vi "HOLD.vi"() -> ()   [LabVIEW 2015]
uses:
  Global.vi
panel:
  out "Options":string
  in  "Hold":bool
  in  "stop":bool
  out "VAR index":i32
  out "Val":string
  out "Old_Val":string
  out "Set":bool
  out "Recieved":bool
  in  "Var":string="HOLD"
  # "Wait for user input.\n\nValue Type: STR\nOptions: None"
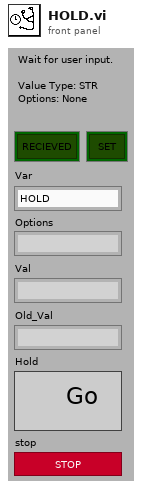
[diagram p1: front panel]
types:
  T1 = typedef "Semaphore RefNum" = refnum<k1>
  T2 = cluster{"VAR":string, "Options":string, "Val":string, "Recieved":bool, "Set":bool}[]
  T3 = cluster{"VAR":string, "Options":string, "Val":string, "Recieved":bool, "Set":bool}
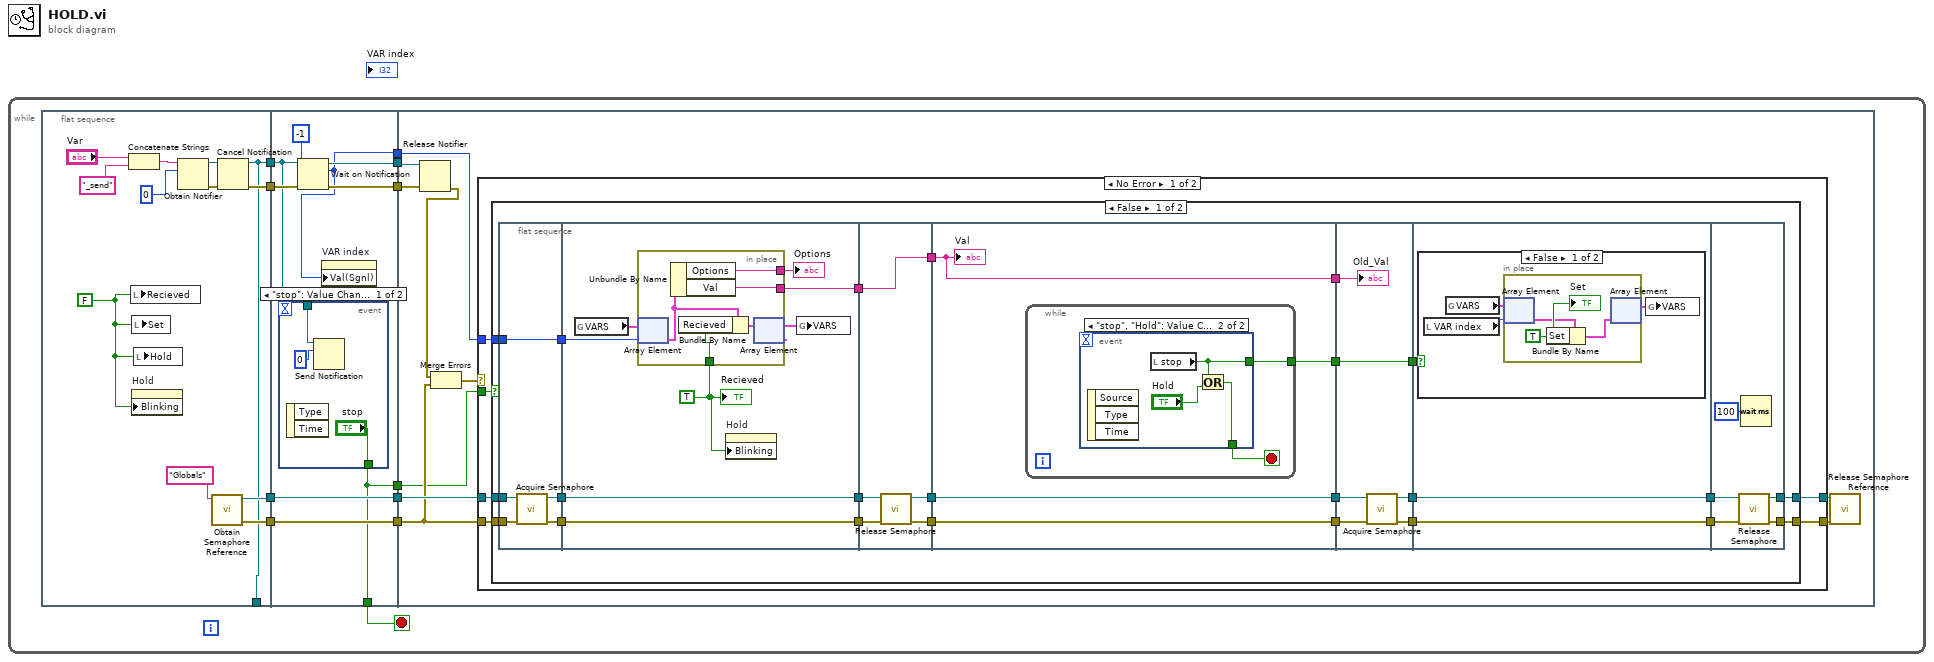
[diagram p0: block diagram]
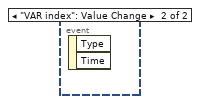
[diagram p2: hidden frame]
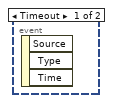
[diagram p3: hidden frame]
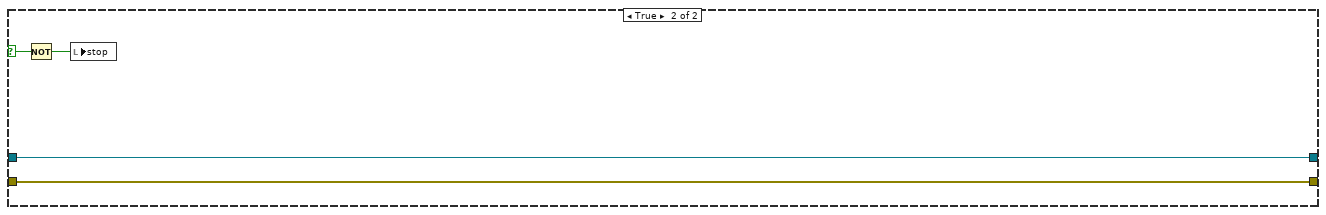
[diagram p5: hidden frame]
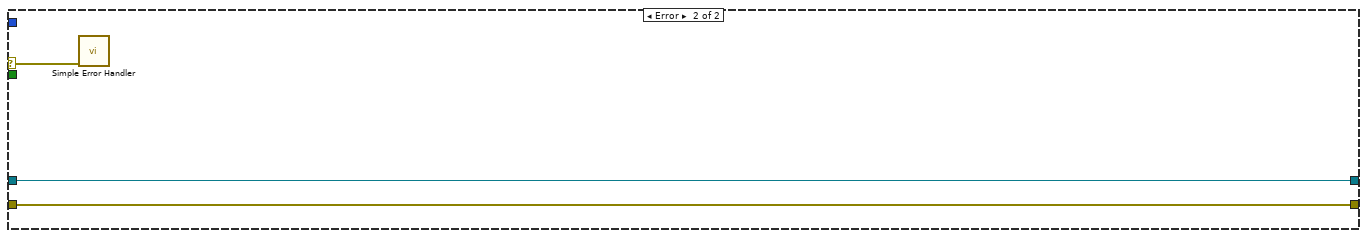
[diagram p6: hidden frame]
diagram:
  n1 = while {
    stop <- w2 stop-if-true
    n2 = flat-sequence {
      tunnel: [w14] -> w11
      tunnel: [w13] -> w10
      tunnel: [w22] -> w6
      tunnel: [w21] -> w4
      tunnel: [w13] -> _
      tunnel: w11 -> [w31]
      tunnel: w10 -> [w25]
      tunnel: [w30] -> w9
      tunnel: [w27] -> w8
      tunnel: [w26] -> w7
      tunnel: w6 -> [w29]
      tunnel: [w29] -> w5
      tunnel: w4 -> [w28]
      tunnel: [w28] -> w3
      tunnel: [w24] -> w2
      tunnel: [w24] -> w1
      tunnel: w9 -> [w38]
      tunnel: w8 -> [w39]
      tunnel: w7 -> [w45]
      tunnel: w5 -> [w44]
      tunnel: w3 -> [w41]
      tunnel: w1 -> [w36]
      frame #0 {
        w16 = FALSE ("notification")
        n3 = Concatenate Strings("Var", "_send") -> (w19:string)
        n4 = local write "Recieved"(w16) -> ()
        n5 = local write "Set"(w16) -> ()
        n6 = property on="Hold" class="Bool (strict)"("Blinking"=w16) -> ()  [unwired: 2 in, 2 out]
        n7 = local write "Hold"(w16) -> ()
        n8 = Obtain Notifier(name (unnamed)=w19, notification data type=0) -> (notifier out=w12:refnum<notifier>, error out=w15:errorcluster)  [unwired: 2 in, 1 out]
        n9 = call <vilib>:"Obtain Semaphore Reference.vi"("name (unnamed)"="Globals") -> ("error out"=w21:errorcluster, "semaphore"=w22:T1)  [unwired: 4 in, 1 out]
        n10 = Cancel Notification(0:w12, 3:w15) -> (8:w13:refnum<notifier>, 11:w14:errorcluster)  [unwired: 1 out]
      }
      frame #1 {
        n11 = event shown="[0] \"stop\": Value Change" {
          selector: _ -> [_ _]
          dyn-events: _ -> [_ _]
          timeout: _ -> [_ _]
          tunnel: ["stop" _] -> w24
          tunnel: w25 -> [w34 _]
          event "stop": Value Change {
            n12 = event-data() -> ()  [unwired: 1 in, 2 out]
            n13 = Send Notification(notification=0, notifier=w34) -> ()  [unwired: 1 in, 2 out]
          }
          event "VAR index": Value Change {
            n14 = event-data() -> ()  [unwired: 1 in, 2 out]
          }
        }
        n15 = Wait on Notification(notifier=w25, timeout in ms (-1)=-1, error in (no error)=w31) -> (notifier out=w30:refnum<notifier>, notification=w26:i32, error out=w27:errorcluster)  [unwired: 1 in, 1 out]
        n16 = property on="VAR index" class="DigNum (strict)"("Val(Sgnl)"=w26) -> ()  [unwired: 2 in, 2 out]
      }
      frame #2 {
        n17 = Release Notifier(notifier=w38, error in (no error)=w39) -> (error out=w37:errorcluster)  [unwired: 1 in, 2 out]
        n18 = Merge Errors(w37, w41) -> (w40:errorcluster)
        n19 = case shown="No Error" w40 {
          selector: w40 -> [_ w131]
          tunnel: w45 -> [w51 _]
          tunnel: w44 -> [w50 w133]
          tunnel: w41 -> [w49 w132]
          tunnel: [w48 w132] -> w43
          tunnel: [w47 w133] -> w42
          tunnel: w36 -> [w46 _]
          frame No Error {
            n20 = case shown="False" w46 {
              selector: w46 -> [_ w128]
              tunnel: w51 -> [w59 _]
              tunnel: w50 -> [w58 w130]
              tunnel: w49 -> [w57 w129]
              tunnel: [w56 w129] -> w48
              tunnel: [w55 w130] -> w47
              frame False {
                n21 = flat-sequence {
                  tunnel: w57 -> [w77]
                  tunnel: w58 -> [w78]
                  tunnel: w59 -> [w79]
                  tunnel: [w79] -> w74
                  tunnel: [w76] -> w73
                  tunnel: [w75] -> w72
                  tunnel: w74 -> [w83]
                  tunnel: w73 -> [w86]
                  tunnel: w72 -> [w87]
                  tunnel: [w87] -> w71
                  tunnel: [w86] -> w70
                  tunnel: [w82] -> w69
                  tunnel: w71 -> [w96]
                  tunnel: w70 -> [w97]
                  tunnel: [w95] -> w68
                  tunnel: [w94] -> w67
                  tunnel: [w93] -> w66
                  tunnel: w69 -> [w93]
                  tunnel: w68 -> [w101]
                  tunnel: w67 -> [w100]
                  tunnel: [w101] -> w65
                  tunnel: [w100] -> w64
                  tunnel: w66 -> [w98]
                  tunnel: [w99] -> w53
                  tunnel: [w98] -> w52
                  tunnel: w65 -> [w112]
                  tunnel: w64 -> [w109]
                  tunnel: [w111] -> w63
                  tunnel: [w110] -> w62
                  tunnel: [w108] -> w54
                  tunnel: w53 -> [w108]
                  tunnel: w52 -> [w107]
                  tunnel: [w115] -> w61
                  tunnel: w63 -> [w115]
                  tunnel: [w114] -> w60
                  tunnel: w62 -> [w114]
                  tunnel: w54 -> [w113]
                  tunnel: w61 -> [w126]
                  tunnel: w60 -> [w125]
                  tunnel: [w124] -> w56
                  tunnel: [w123] -> w55
                  frame #0 {
                    n22 = call <vilib>:"Acquire Semaphore.vi"("error in (no error)"=w77, "semaphore"=w78) -> ("error out"=w76:errorcluster, "semaphore out"=w75:T1)  [unwired: 3 in, 1 out]
                  }
                  frame #1 {
                    w81 = TRUE ("Found")
                    n23 = global read "Global.vi" "VARS"() -> (w84:T2)
                    n24 = in-place {
                      in-place-border: [w90] -> w82
                      in-place-border: w81 -> [w89]
                      in-place-border: [w88] -> w80
                      n25 = in-place-array #1(w84, w83) -> (w92:T3)
                      n26 = Unbundle By Name(w92) -> ("Options"=w88:string, "Val"=w90:string)
                      n27 = Bundle By Name(cluster=w92, "Recieved"=w89) -> (w91:T3)
                      n28 = in-place-array #1(w91) -> (w85:T2)  [unwired: 1 out]
                    }
                    "Options" <- w80
                    n29 = property on="Hold" class="Bool (strict)"("Blinking"=w81) -> ()  [unwired: 2 in, 2 out]
                    n30 = global write "Global.vi" "VARS"(w85) -> ()
                    "Recieved" <- w81
                  }
                  frame #2 {
                    n31 = call <vilib>:"Release Semaphore.vi"("error in (no error)"=w97, "semaphore"=w96) -> ("error out"=w94:errorcluster, "semaphore out"=w95:T1)  [unwired: 4 in]
                  }
                  frame #3 {
                    n32 = while {
                      tunnel: [w102] -> w99
                      stop <- w103 stop-if-true
                      n33 = event shown="[1] \"stop\", \"Hold\": Value Change" {
                        selector: _ -> [_ _]
                        dyn-events: _ -> [_ _]
                        timeout: _ -> [_ _]
                        tunnel: [_ w105] -> w103
                        tunnel: [_ w104] -> w102
                        event Timeout {
                          n34 = event-data() -> ()  [unwired: 1 in, 3 out]
                        }
                        event "stop", "Hold": Value Change {
                          n35 = event-data() -> ()  [unwired: 1 in, 3 out]
                          n36 = local read "stop"() -> (w104:bool)
                          n37 = Or(x=w104, y="Hold") -> (x .or. y?=w105:bool)
                        }
                      }
                    }
                    "Val" <- w98
                  }
                  frame #4 {
                    n38 = call <vilib>:"Acquire Semaphore.vi"("error in (no error)"=w109, "semaphore"=w112) -> ("error out"=w110:errorcluster, "semaphore out"=w111:T1)  [unwired: 3 in, 1 out]
                    "Old_Val" <- w107
                  }
                  frame #5 {
                    n39 = case shown="False" w113 {
                      frame False {
                        n40 = local read "VAR index"() -> (w118:i32)
                        n41 = global read "Global.vi" "VARS"() -> (w117:T2)
                        n42 = in-place {
                          w121 = TRUE ("Set")
                          n43 = in-place-array #2(w117, w118) -> (w120:T3)
                          n44 = Bundle By Name(cluster=w120, "Set"=w121) -> (w119:T3)
                          n45 = in-place-array #2(w119) -> (w116:T2)  [unwired: 1 out]
                          "Set" <- w121
                        }
                        n46 = global write "Global.vi" "VARS"(w116) -> ()
                      }
                      frame True {
                      }
                    }
                  }
                  frame #6 {
                    n47 = call <vilib>:"Release Semaphore.vi"("error in (no error)"=w125, "semaphore"=w126) -> ("error out"=w124:errorcluster, "semaphore out"=w123:T1)  [unwired: 4 in]
                    n48 = Wait (ms)(milliseconds to wait=u32 100) -> ()  [unwired: 1 out]
                  }
                }
              }
              frame True {
                n49 = Not(x=w128) -> (.not. x?=w127:bool)
                n50 = local write "stop"(w127) -> ()
              }
            }
          }
          frame Error {
            n51 = call <vilib>:"Simple Error Handler.vi"("error in (no error)"=w131) -> ()  [unwired: 4 in, 5 out]
          }
        }
        n52 = call <vilib>:"Release Semaphore Reference.vi"("error in (no error)"=w43, "semaphore"=w42) -> ()  [unwired: 8 in, 2 out]
      }
    }
  }
